vi "GetControlTerminalReference.vi"(0 "Control Terminal References":T1[](array[typedef]), 5 "Control Name":string) -> (4 "Terminal Reference":refnum<vi>)   [LabVIEW 2019, in "JsonToCluster.lvlib"]
doc: "This VI gets required control terminal reference to connect with Unflatten from JSON string"
uses:
  JsonToCluster.lvlib
  _Controls/ControlTerminalReference.ctl
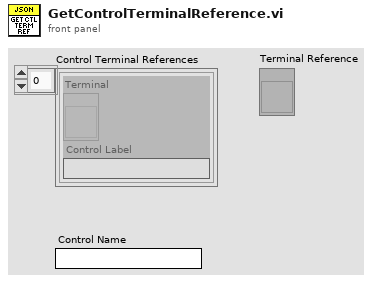
[diagram p1: front panel]
types:
  T1 = typedef "JsonToCluster.lvlib/ControlTerminalReference.ctl" = cluster{"Terminal":refnum<vi>, "Control Label":string}
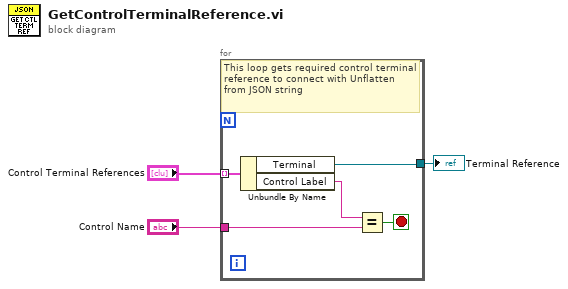
[diagram p0: block diagram]
diagram:
  n1 = for {
    tunnel: "Control Terminal References" -> [w8] mode=indexing
    tunnel: "Control Name" -> [w6]
    tunnel: [w4] -> w1
    stop <- w5 stop-if-true
    # "This loop gets required control terminal reference to connect with Unflatten from JSON string"
    n2 = Unbundle By Name(w8) -> ("Terminal"=w4:refnum<vi>, "Control Label"=w7:string)
    n3 = Equal?(x=w7, y=w6) -> (x = y?=w5:bool)
  }
  "Terminal Reference" <- w1
